vi "sub_main_erp42.vi"(8 "error in":errorcluster) -> (0 "error out":errorcluster)   [LabVIEW 2019]
uses:
  Ctrl/data.ctl
panel:
  out "count":i32
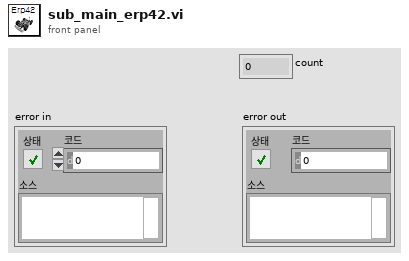
[diagram p1: front panel]
types:
  T1 = typedef "data.ctl" = cluster{"Drive_value":cluster{"F/B":enum16{"Go", "N", "Back"}, "Speed":u16, "Steer":i16, "A/M":enum16{"Brake", "Auto", "Manual"}, "Brake":u8}}
  T2 = typedef "status.ctl" = u16
  T3 = cluster{"AGV":T2, "AGV Estop":T2, "Obstacle":T2, "Heading":T2, "Waypt":T2, "GNSS":T2, "VLP16":T2, "Cam":T2, "RPLidar":T2, "Joystick":T2}
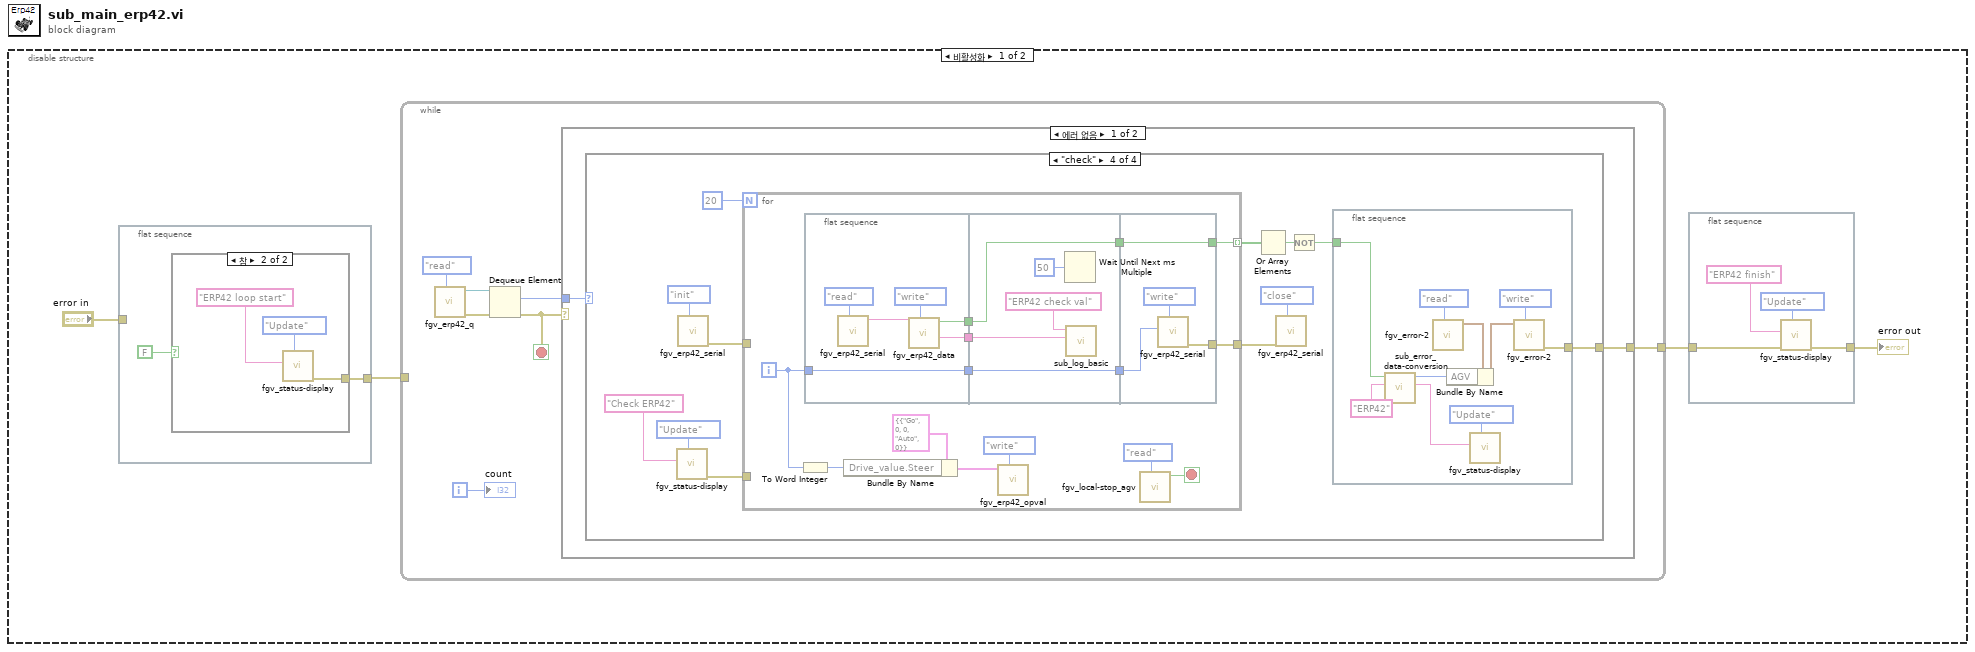
[diagram p0: block diagram]
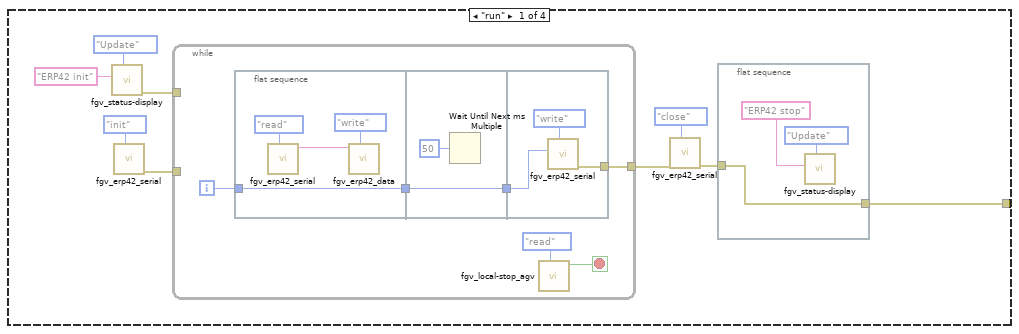
[diagram p3: hidden frame]
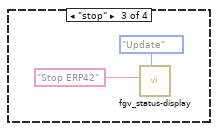
[diagram p5: hidden frame]
diagram:
  n1 = disable-structure shown="비활성화" {
    frame Disabled {
      n2 = flat-sequence {
        tunnel: [w10] -> w1
        tunnel: "error in" -> [_]
        frame #0 {
          n3 = case shown="참" FALSE {
            tunnel: [_ w11] -> w10
            frame False {
            }
            frame True {
              n4 = call "fgv_status-display.vi"("Mode"=enum16{"Initial", "Update", "Clear"}."Update", "title"="ERP42 loop start" ("String in 1")) -> ("error out"=w11:errorcluster)  [unwired: 9 in]
            }
          }
        }
      }
      n5 = while {
        tunnel: w1 -> [_]
        tunnel: [w16] -> w2
        i -> [w15]
        stop <- w14 stop-if-true
        n6 = call "fgv_erp42_q.vi"("cmd"=enum16{"create", "write", "read", "close"}."read") -> ("error out"=w18:errorcluster, "queue out"=w19:refnum<queue>)  [unwired: 9 in]
        n7 = Dequeue Element(queue=w19, error in (no error)=w18) -> (element=w17:enum16{"run", "check", "stop"}, error out=w14:errorcluster)  [unwired: 1 in, 2 out]
        n8 = case shown="에러 없음" w14 {
          tunnel: w17 -> [w22 _]
          tunnel: [w21 _] -> w16
          frame No Error {
            n9 = case shown="\"check\"" w22 {
              tunnel: [w27 _ _ w52] -> w21
              frame "run" {
                n10 = call "fgv_status-display.vi"("Mode"=enum16{"Initial", "Update", "Clear"}."Update", "title"="ERP42 init") -> ("error out"=w23:errorcluster)  [unwired: 9 in]
                n11 = call "fgv_erp42_serial.vi"("cmd"=enum16{"init", "read", "write", "close"}."init") -> ("error out"=w25:errorcluster)  [unwired: 7 in, 3 out]
                n12 = while {
                  tunnel: w25 -> [_]
                  tunnel: [w35] -> w29
                  tunnel: w23 -> [_]
                  i -> [w38]
                  stop <- w36 stop-if-true
                  n13 = flat-sequence {
                    tunnel: [w43] -> w39
                    tunnel: w38 -> [w43]
                    tunnel: [w45] -> w40
                    tunnel: w39 -> [w45]
                    tunnel: w40 -> [w48]
                    tunnel: [w47] -> w35
                    frame #0 {
                      n14 = call "fgv_erp42_serial.vi"("cmd"=enum16{"init", "read", "write", "close"}."read") -> ("read_buffer"=w42:string)  [unwired: 7 in, 3 out]
                      n15 = call "fgv_erp42_data.vi"("cmd"=enum16{"init", "read", "write"}."write", "erp recv str"=w42) -> ()  [unwired: 7 in, 3 out]
                    }
                    frame #1 {
                      n16 = Wait Until Next ms Multiple(millisecond multiple=u32 50 ("ms 배수")) -> ()  [unwired: 1 out]
                    }
                    frame #2 {
                      n17 = call "fgv_erp42_serial.vi"("cmd"=enum16{"init", "read", "write", "close"}."write", "count"=w48) -> ("error out"=w47:errorcluster)  [unwired: 6 in, 3 out]
                    }
                  }
                  n18 = call "fgv_local-stop_agv.vi"("cmd"=enum16{"ini", "read", "stop"}."read") -> ("stop status"=w36:bool)  [unwired: 10 in]
                }
                n19 = call "fgv_erp42_serial.vi"("cmd"=enum16{"init", "read", "write", "close"}."close", "error in"=w29) -> ("error out"=w28:errorcluster)  [unwired: 6 in, 3 out]
                n20 = flat-sequence {
                  tunnel: w28 -> [w34]
                  tunnel: [w34] -> w27
                  frame #0 {
                    n21 = call "fgv_status-display.vi"("Mode"=enum16{"Initial", "Update", "Clear"}."Update", "title"="ERP42 stop" ("String in 1")) -> ()  [unwired: 9 in, 1 out]
                  }
                }
              }
              frame Default {
              }
              frame "stop" {
                n22 = call "fgv_status-display.vi"("Mode"=enum16{"Initial", "Update", "Clear"}."Update", "title"="Stop ERP42" ("String in")) -> ()  [unwired: 9 in, 1 out]
              }
              frame "check" {
                n23 = call "fgv_status-display.vi"("Mode"=enum16{"Initial", "Update", "Clear"}."Update", "title"="Check ERP42" ("String in")) -> ("error out"=w53:errorcluster)  [unwired: 9 in]
                n24 = call "fgv_erp42_serial.vi"("cmd"=enum16{"init", "read", "write", "close"}."init") -> ("error out"=w60:errorcluster)  [unwired: 7 in, 3 out]
                n25 = for {
                  N: 20 -> [_]
                  tunnel: w60 -> [_]
                  tunnel: [w84] -> w61
                  tunnel: [w82] -> w54 mode=indexing
                  tunnel: w53 -> [_]
                  i -> [w76]
                  stop <- w83 stop-if-true
                  n26 = To Word Integer(number=w76) -> (16bit integer=w75:i16)
                  n27 = flat-sequence {
                    tunnel: [w92] -> w86
                    tunnel: w76 -> [w92]
                    tunnel: [w89] -> w80
                    tunnel: [w88] -> w74
                    tunnel: [w97] -> w87
                    tunnel: w86 -> [w97]
                    tunnel: [w96] -> w81
                    tunnel: w80 -> [w96]
                    tunnel: w74 -> [w94]
                    tunnel: w87 -> [w101]
                    tunnel: [w100] -> w84
                    tunnel: [w99] -> w82
                    tunnel: w81 -> [w99]
                    frame #0 {
                      n28 = call "fgv_erp42_serial.vi"("cmd"=enum16{"init", "read", "write", "close"}."read") -> ("read_buffer"=w90:string)  [unwired: 7 in, 3 out]
                      n29 = call "fgv_erp42_data.vi"("cmd"=enum16{"init", "read", "write"}."write", "erp recv str"=w90) -> ("erp recv out"=w88:string, "val"=w89:bool)  [unwired: 7 in, 1 out]
                    }
                    frame #1 {
                      n30 = Wait Until Next ms Multiple(millisecond multiple=u32 50 ("ms 배수")) -> ()  [unwired: 1 out]
                      n31 = call "sub_log_basic.vi"("desc"=w94, "Title"="ERP42 check val") -> ()  [unwired: 9 in, 1 out]
                    }
                    frame #2 {
                      n32 = call "fgv_erp42_serial.vi"("cmd"=enum16{"init", "read", "write", "close"}."write", "count"=w101) -> ("error out"=w100:errorcluster)  [unwired: 6 in, 3 out]
                    }
                  }
                  n33 = Bundle By Name(cluster=T1 {"Drive_value"={"F/B"=enum."Go", "Speed"=0, "Steer"=0, "A/M"=enum."Auto", "Brake"=0}} ("data_in"), "Drive_value.Steer"=w75) -> (w77:T1)
                  n34 = call "fgv_erp42_opval.vi"("cmd"=enum16{"read", "write", "ini"}."write", "data_in"=w77) -> ()  [unwired: 9 in, 1 out]
                  n35 = call "fgv_local-stop_agv.vi"("cmd"=enum16{"ini", "read", "stop"}."read") -> ("stop status"=w83:bool)  [unwired: 10 in]
                }
                n36 = Or Array Elements(Boolean array=w54) -> (logical OR=w56:bool)
                n37 = call "fgv_erp42_serial.vi"("cmd"=enum16{"init", "read", "write", "close"}."close", "error in"=w61) -> ()  [unwired: 6 in, 4 out]
                n38 = Not(x=w56) -> (.not. x?=w55:bool)
                n39 = flat-sequence {
                  tunnel: w55 -> [w68]
                  tunnel: [w64] -> w52
                  frame #0 {
                    n40 = call "sub_error_data-conversion.vi"("name"="ERP42", "error status"=w68) -> ("check result string"=w66:string, "error conversion out"=w73:T2)  [unwired: 8 in]
                    n41 = call "fgv_error-2.vi"("cmd"=enum16{"init", "read", "write"}."read") -> ("Error cluster out"=w72:T3)  [unwired: 9 in, 1 out]
                    n42 = Bundle By Name(cluster=w72, "AGV"=w73) -> (w71:T3)
                    n43 = call "fgv_status-display.vi"("Mode"=enum16{"Initial", "Update", "Clear"}."Update", "title"=w66) -> ()  [unwired: 9 in, 1 out]
                    n44 = call "fgv_error-2.vi"("cmd"=enum16{"init", "read", "write"}."write", "Error cluster"=w71) -> ("error out"=w64:errorcluster)  [unwired: 8 in, 1 out]
                  }
                }
              }
            }
          }
          frame Error {
          }
        }
        "count" <- w15
      }
      n45 = flat-sequence {
        tunnel: [w6] -> w3
        tunnel: w2 -> [w5]
        frame #0 {
          n46 = call "fgv_status-display.vi"("Mode"=enum16{"Initial", "Update", "Clear"}."Update", "error in"=w5, "title"="ERP42 finish" ("String in 1")) -> ("error out"=w6:errorcluster)  [unwired: 8 in]
        }
      }
      "error out" <- w3
    }
    frame Enabled {
    }
  }
